vi "filterPortionTrajectories.vi"(8 "error in (no error)":errorcluster, 9 "ToHoloN°":u32, 10 "FromHoloN°":u32, 11 "AllTrajectories in":dbl[][](array[numeric])) -> (0 "error out":errorcluster, 3 "AllTrajectories out":dbl[][](array[numeric]))   [LabVIEW 2023]
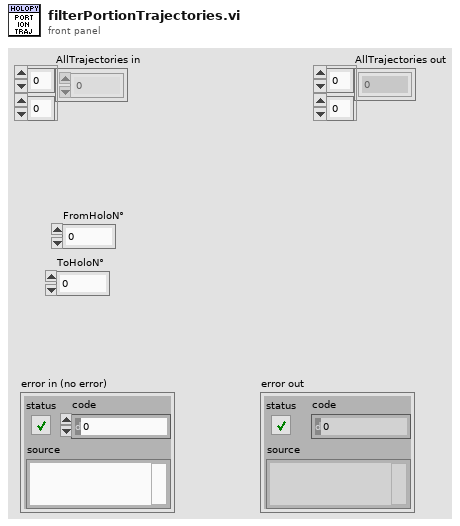
[diagram p1: front panel]
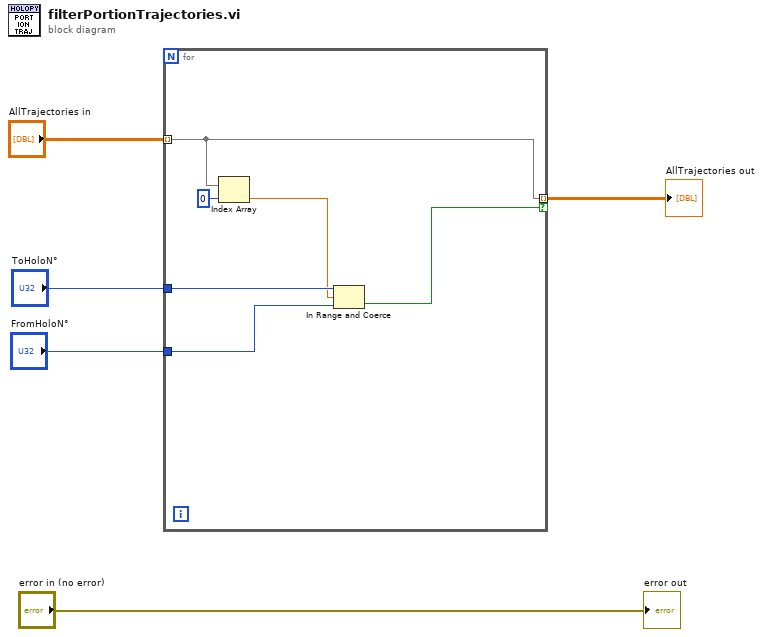
[diagram p0: block diagram]
diagram:
  n1 = for {
    tunnel: "AllTrajectories in" -> [w6] mode=indexing
    tunnel: "ToHoloN°" -> [w10]
    tunnel: "FromHoloN°" -> [w9]
    tunnel: [w6] -> w1 mode=indexing if=w7
    n2 = Index Array(array=w6, index=0) -> (element=w8:dbl)
    n3 = In Range and Coerce(upper limit=w10, x=w8, lower limit=w9) -> (In Range?=w7:bool)  [unwired: 1 out]
  }
  "AllTrajectories out" <- w1
  "error out" <- "error in (no error)"
